vi "Channel2Board.vi"(11 "channel":u8) -> (3 "Numeric":u8)   [LabVIEW 2016]
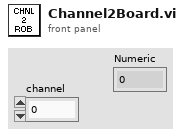
[diagram p1: front panel]
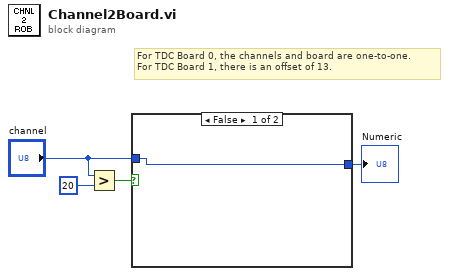
[diagram p0: block diagram]
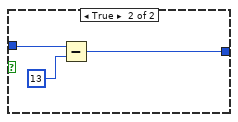
[diagram p2: hidden frame]
diagram:
  # "For TDC Board 0, the channels and board are one-to-one.\nFor TDC Board 1, there is an offset of 13."
  n1 = Greater?(x="channel", y=u8 20) -> (0:w3:bool)
  n2 = case shown="False" w3 {
    tunnel: "channel" -> [w5 w8]
    tunnel: [w5 w6] -> w1
    frame False {
    }
    frame True {
      n3 = Subtract(x=w8, y=u8 13) -> (x-y=w6:u8)
    }
  }
  "Numeric" <- w1
